vi "VTx_control_Juniper.vi"(4 "VTx_Voltage":dbl, 6 "VTxIndex_In":i8, 8 "error in (no error)":errorcluster, 9 "VTx1_voltage":dbl, 10 "Timeout (ms)":i32=40000000, 11 "connection ID in":refnum<k5>) -> (0 "error out":errorcluster, 3 "connection ID out":refnum<k5>)   [LabVIEW 2016]
uses:
  TemperatureMeasure/Thermal_type.vi
panel:
  out "check_VTx0":dbl
  out "check_VTx1":dbl
  out "Bigger?":bool
  out "Read_VTx1":dbl
  out "Read_VTx0":dbl
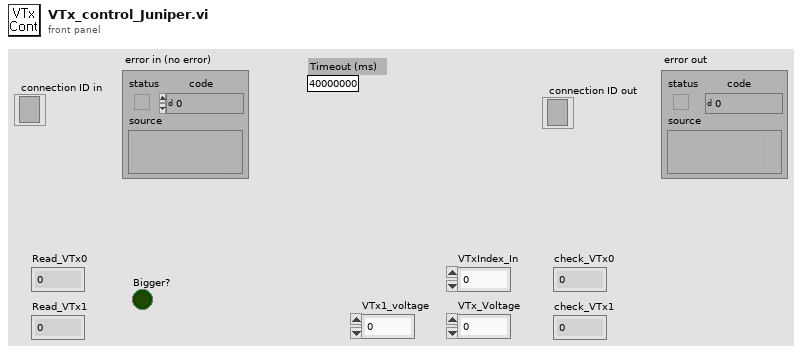
[diagram p1: front panel]
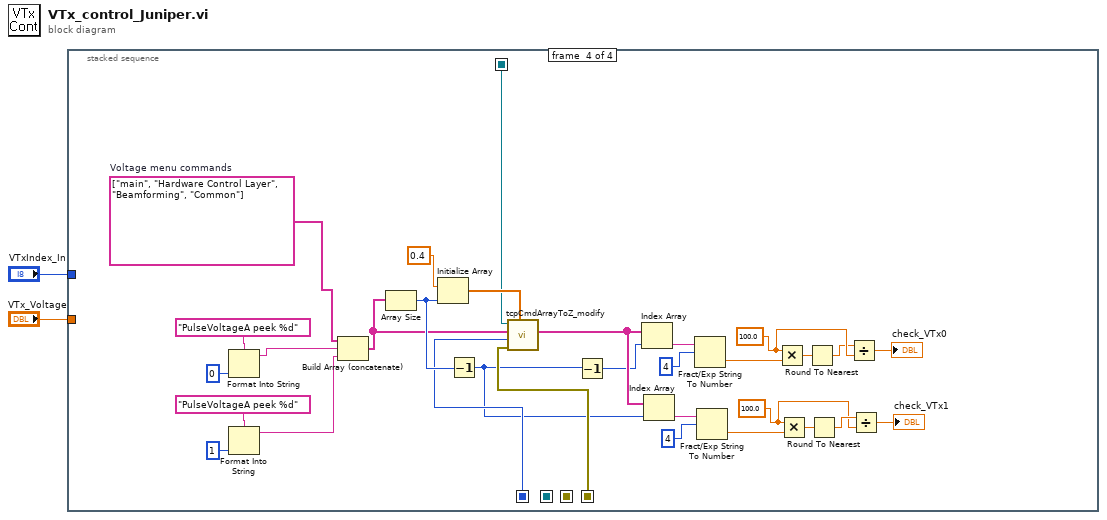
[diagram p0: block diagram]
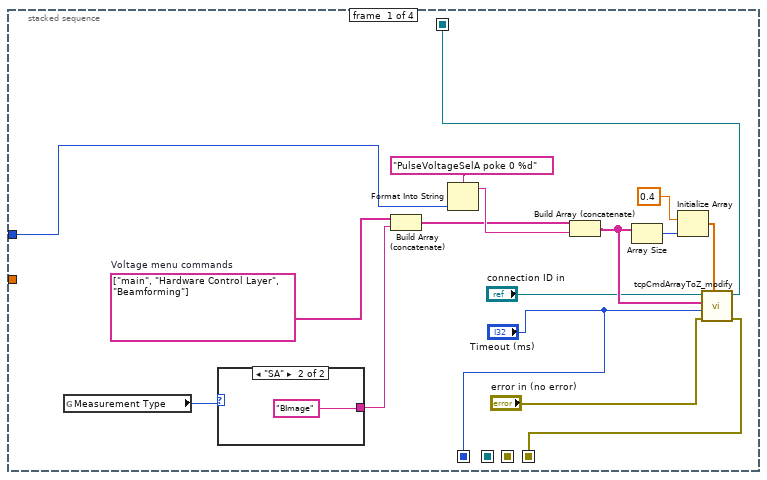
[diagram p2: hidden frame]
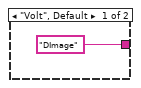
[diagram p3: hidden frame]
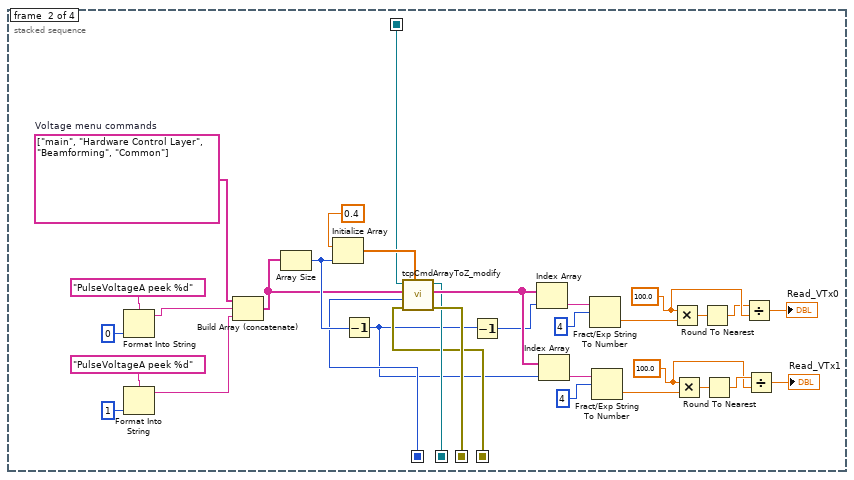
[diagram p4: hidden frame]
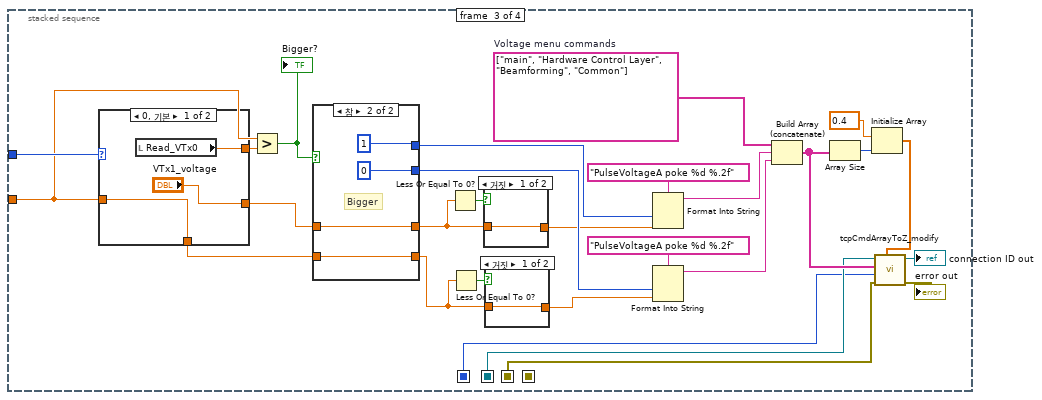
[diagram p5: hidden frame]
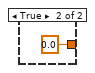
[diagram p6: hidden frame]
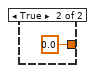
[diagram p7: hidden frame]
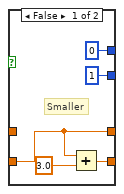
[diagram p8: hidden frame]
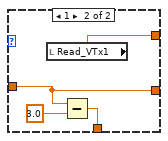
[diagram p9: hidden frame]
diagram:
  n1 = stacked-sequence {
    seq-local: [_ w28 _ _] -> [_ _ w65 _]
    seq-local: [_ w27 _ _] -> [_ _ w66 _]
    seq-local: ["Timeout (ms)" _ _ _] -> [_ w26 w64 w107]
    seq-local: [w5 _ _ _] -> [_ w25 _ w106]
    seq-local: [w4 _ _ _] -> [_ w24 _ w105]
    tunnel: "VTxIndex_In" -> [w13 _ w80 _]
    tunnel: "VTx_Voltage" -> [_ _ w69 _]
    frame #0 {
      w3 = string[] ["main", "Hardware Control Layer", "Beamforming"]  # Voltage menu commands
      n2 = global read "Thermal_type.vi" "Measurement Type"() -> (w18:enum32{"Volt", "SA"})
      n3 = case shown="\"SA\"" w18 {
        tunnel: ["DImage" "BImage"] -> w17
        frame "Volt", Default {
        }
        frame "SA" {
        }
      }
      n4 = Build Array (concatenate)(w3, w17) -> (w14:string[])
      n5 = Format Into String(format string="PulseVoltageSelA poke 0 %d" ("포맷 문자열"), w13) -> (resulting string=w15:string)  [unwired: 2 in, 1 out]
      n6 = Build Array (concatenate)(w14, w15) -> (w9:string[])
      n7 = Array Size(array=w9) -> (size(s)=w12:i32)
      n8 = Initialize Array(0.4 ("원소"), w12) -> (w10:dbl[])
      n9 = call "tcpCmdArrayToZ_modify.vi"("Delay (sec)"=w10, "error in (no error)"="error in (no error)", "Timeout (ms)"="Timeout (ms)", "Command array"=w9, "connection ID in"="connection ID in") -> ("error out"=w5:errorcluster, "connection ID out"=w4:refnum<k5>)  [unwired: 2 in, 3 out]
    }
    frame #1 {
      w21 = string[] ["main", "Hardware Control Layer", "Beamforming", "Common"]  # Voltage menu commands
      w35 = 100.0
      w47 = 100.0
      n10 = Format Into String(format string="PulseVoltageA peek %d", i8 0 ("입력 1")) -> (resulting string=w41:string)  [unwired: 2 in, 1 out]
      n11 = Format Into String(format string="PulseVoltageA peek %d", i8 1 ("입력 1")) -> (resulting string=w38:string)  [unwired: 2 in, 1 out]
      n12 = Build Array (concatenate)(w21, w41, w38) -> (w43:string[])
      n13 = Array Size(array=w43) -> (size(s)=w51:i32)
      n14 = Initialize Array(0.4 ("원소"), w51) -> (w52:dbl[])
      n15 = Decrement(x=w51) -> (x-1=w22:i32)
      n16 = call "tcpCmdArrayToZ_modify.vi"("Delay (sec)"=w52, "error in (no error)"=w25, "Timeout (ms)"=w26, "Command array"=w43, "connection ID in"=w24) -> ("error out"=w28:errorcluster, "Receive array"=w31:string[], "connection ID out"=w27:refnum<k5>)  [unwired: 2 in, 2 out]
      n17 = Decrement(x=w22) -> (x-1=w23:i32)
      n18 = Index Array(array=w31, index=w23) -> (element=w50:string)
      n19 = Index Array(array=w31, index=w22) -> (element=w32:string)
      n20 = Fract/Exp String To Number(string=w50, offset=4 ("오프셋")) -> (number=w45:dbl)  [unwired: 2 in, 1 out]
      n21 = Fract/Exp String To Number(string=w32, offset=4 ("오프셋")) -> (number=w37:dbl)  [unwired: 2 in, 1 out]
      n22 = Multiply(x=w47, y=w45) -> (x*y=w48:dbl)
      n23 = Multiply(x=w35, y=w37) -> (x*y=w34:dbl)
      n24 = Round To Nearest(number=w48) -> (nearest integer value=w46:dbl)
      n25 = Round To Nearest(number=w34) -> (nearest integer value=w36:dbl)
      n26 = Divide(x=w46, y=w47) -> (x/y=→"Read_VTx0":dbl)
      n27 = Divide(x=w36, y=w35) -> (x/y=→"Read_VTx1":dbl)
    }
    frame #2 {
      w54 = string[] ["main", "Hardware Control Layer", "Beamforming", "Common"]  # Voltage menu commands
      n28 = case shown="0, 기본" w80 {
        tunnel: [w97 w101] -> w81
        tunnel: ["VTx1_voltage" w99] -> w68
        tunnel: [w96 w100] -> w67
        tunnel: w69 -> [w96 w99]
        frame 0, Default {
          n29 = local read "Read_VTx0"() -> (w97:dbl)
        }
        frame 1 {
          n30 = local read "Read_VTx1"() -> (w101:dbl)
          n31 = Subtract(x=w99, y=3.0) -> (x-y=w100:dbl)
        }
      }
      n32 = Greater?(x=w69, y=w81) -> (0:w72:bool)
      "Bigger?" <- w72
      n33 = case shown="참" w72 {
        tunnel: [0 1] -> w71
        tunnel: [1 0] -> w70
        tunnel: [w86 w92] -> w59
        tunnel: w68 -> [_ w92]
        tunnel: w67 -> [w86 w91]
        tunnel: [w87 w91] -> w56
        frame False {
          # "Smaller"
          n34 = Add(x=w86, y=3.0) -> (x+y=w87:dbl)
        }
        frame True {
          # "Bigger"
        }
      }
      n35 = Less Or Equal To 0?(x=w59) -> (x <= 0?=w60:bool)
      n36 = Less Or Equal To 0?(x=w56) -> (x <= 0?=w57:bool)
      n37 = case shown="거짓" w60 {
        tunnel: w59 -> [w84 _]
        tunnel: [w84 0.0 ("VTx_Voltage")] -> w58
        frame False {
        }
        frame True {
        }
      }
      n38 = case shown="거짓" w57 {
        tunnel: w56 -> [w82 _]
        tunnel: [w82 0.0 ("VTx_Voltage")] -> w55
        frame False {
        }
        frame True {
        }
      }
      n39 = Format Into String(format string="PulseVoltageA poke %d %.2f" ("Format String"), w71, w58) -> (resulting string=w75:string)  [unwired: 2 in, 1 out]
      n40 = Format Into String(format string="PulseVoltageA poke %d %.2f" ("Format String"), w70, w55) -> (resulting string=w61:string)  [unwired: 2 in, 1 out]
      n41 = Build Array (concatenate)(w54, w75, w61) -> (w79:string[])
      n42 = Array Size(array=w79) -> (size(s)=w76:i32)
      n43 = Initialize Array(0.4 ("element"), w76) -> (w78:dbl[])
      n44 = call "tcpCmdArrayToZ_modify.vi"("Delay (sec)"=w78, "error in (no error)"=w65, "Timeout (ms)"=w64, "Command array"=w79, "connection ID in"=w66) -> ("error out"=→"error out":errorcluster, "connection ID out"=→"connection ID out":refnum<k5>)  [unwired: 2 in, 3 out]
    }
    frame #3 {
      w102 = string[] ["main", "Hardware Control Layer", "Beamforming", "Common"]  # Voltage menu commands
      w114 = 100.0
      w126 = 100.0
      n45 = Format Into String(format string="PulseVoltageA peek %d", i8 0 ("입력 1")) -> (resulting string=w120:string)  [unwired: 2 in, 1 out]
      n46 = Format Into String(format string="PulseVoltageA peek %d", i8 1 ("입력 1")) -> (resulting string=w117:string)  [unwired: 2 in, 1 out]
      n47 = Build Array (concatenate)(w102, w120, w117) -> (w122:string[])
      n48 = Array Size(array=w122) -> (size(s)=w130:i32)
      n49 = Initialize Array(0.4 ("원소"), w130) -> (w131:dbl[])
      n50 = Decrement(x=w130) -> (x-1=w103:i32)
      n51 = call "tcpCmdArrayToZ_modify.vi"("Delay (sec)"=w131, "error in (no error)"=w106, "Timeout (ms)"=w107, "Command array"=w122, "connection ID in"=w105) -> ("Receive array"=w110:string[])  [unwired: 2 in, 4 out]
      n52 = Decrement(x=w103) -> (x-1=w104:i32)
      n53 = Index Array(array=w110, index=w104) -> (element=w129:string)
      n54 = Index Array(array=w110, index=w103) -> (element=w111:string)
      n55 = Fract/Exp String To Number(string=w129, offset=4 ("오프셋")) -> (number=w124:dbl)  [unwired: 2 in, 1 out]
      n56 = Fract/Exp String To Number(string=w111, offset=4 ("오프셋")) -> (number=w116:dbl)  [unwired: 2 in, 1 out]
      n57 = Multiply(x=w126, y=w124) -> (x*y=w127:dbl)
      n58 = Multiply(x=w114, y=w116) -> (x*y=w113:dbl)
      n59 = Round To Nearest(number=w127) -> (nearest integer value=w125:dbl)
      n60 = Round To Nearest(number=w113) -> (nearest integer value=w115:dbl)
      n61 = Divide(x=w125, y=w126) -> (x/y=→"check_VTx0":dbl)
      n62 = Divide(x=w115, y=w114) -> (x/y=→"check_VTx1":dbl)
    }
  }
